vi "FreqTURBOGraph_ENGULx.vi"(0 "LCR-819 port name":refnum<visa-resource-name>="COM7") -> ()   [LabVIEW 2016]
doc: "The Basic Serial Read and Write example performs a Serial Port Read, a Serial Port Write, or a combination of these actions. The user selects the actions (read or write) on the front panel. If both are selected, the VI will write the data first, read data, and then close the VISA session that is opened to the port. This VI will wait until the specified number of bytes is received at the port. Only the number of bytes specified will be read.\n\nINSTRUCTIONS:\n1) Select the serial resource and configuration parameters (baud rate, data bits, parity, stop bits, flow control).\n2) Select the operations to be performed. \n3) Connect the serial port to your device. If no device is available, perform a loopback test by doing one of the following. Short pins 2 and 3 on a RS-232 cable or short pin 4 to pin 8 and pin 5 to pin 9 on a RS-485/422 cable. \n4) Run the VI to see the data read. (The \"read string\" will match the \"string to write\" if a loopback test was performed.)\n\nNote: The parameters set for the serial port must match the parameters of the connected instrument or device. In this example, the bytes to read parameter specifies the number of bytes that the serial port reads. If there were more bytes at the port than the number specified in bytes to read, those bytes would not be read. Also, if you specify to read more bytes than the number of bytes actually read, you might receive a timeout error message.\n\nOn the block diagram, the Configure Serial Port VI sets the configuration parameters. The front panel displays the controls used to configure the basic parameters, such as baud rate, data bits, and parity. Constants configure the other parameters the user probably does not need set. After the VISA Configure Serial Port VI opens the VISA session and configures the port, the VI passes the VISA resource name to other VIs that perform operations on that VISA resource. The VISA Write function sends a command to the serial device and the VISA Read function returns data based on the command. The VISA Close function then closes the reference to the serial device. It is important to close the reference; otherwise communication through with that port through protocols other than VISA might not be possible."
uses:
  <vilib>/Instr/_visa.llb/VISA Configure Serial Port (Instr).vi
panel:
  in  "STOP":bool
  out "Temperature, К":dbl
  out "Cole-Cole plot":cluster{dbl, dbl}[](graph)
  out "Frequency dependency of E' E\"":cluster{dbl, dbl, dbl}[](graph)
  out "Epsilon\"":dbl
  out "Epsilon'":dbl
  in  "Thickness, mm":dbl=1.75
  in  "Area, mm2":dbl=20.0
  in  "Comments":string="Sn2P2S6HighT\nS=20mm2 D=1.75mm\n"
  out "Data File":path
  in  "File name":path=path "proba.txt"
  out "Frequency, kHz":dbl
  out "Loss":dbl
  out "Capacity, F":dbl
  out "Current Frequency":string
  out "Frequency":string
  out "Data from LCR-meter":string
  out "Output":string
  # "LCR-819 Service information"
  # "Output Data File"
  # "Data from LCR-meter"
  # "Sample Size"
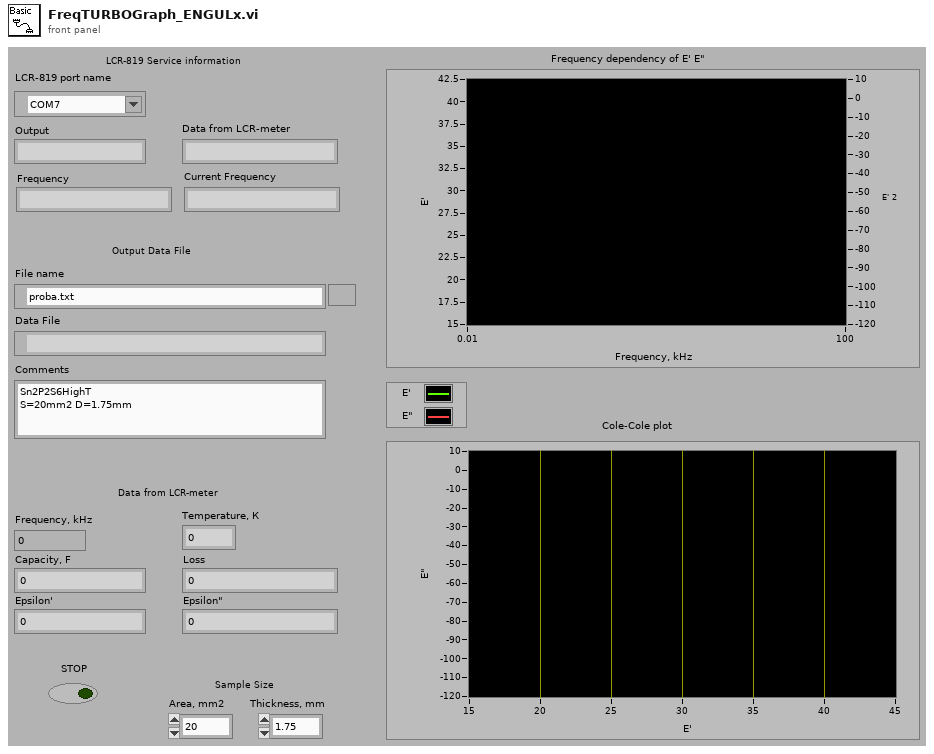
[diagram p1: front panel]
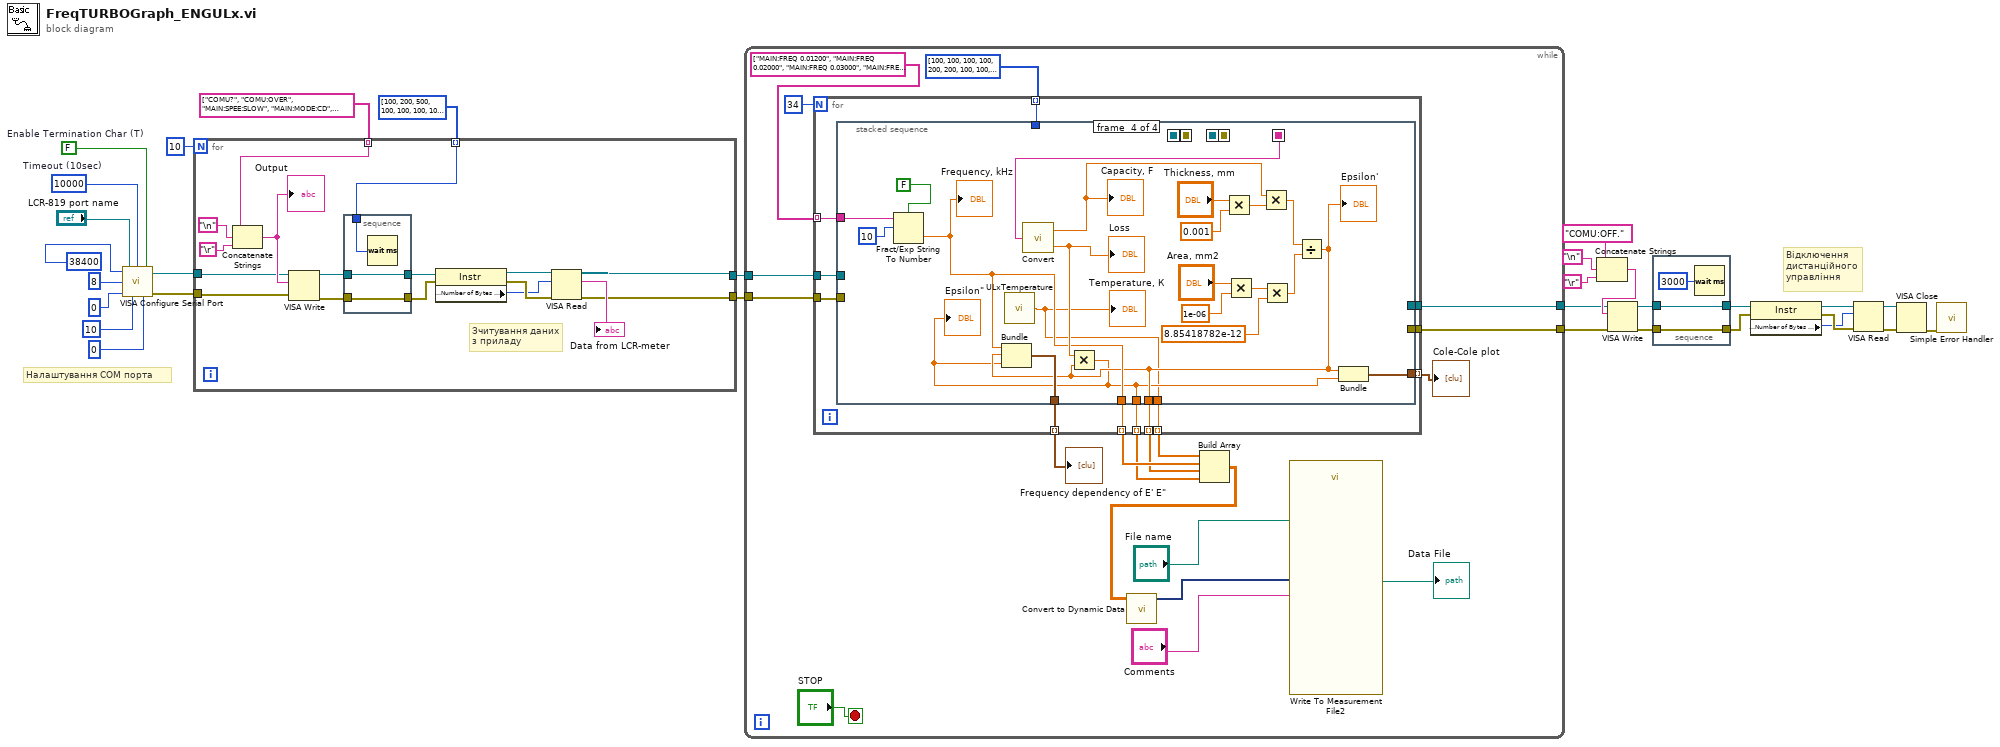
[diagram p0: block diagram]
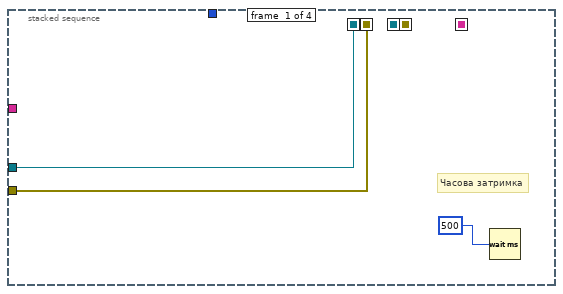
[diagram p2: hidden frame]
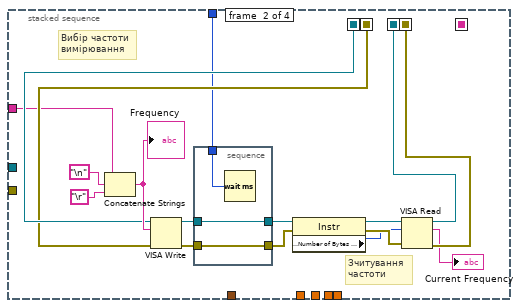
[diagram p3: hidden frame]
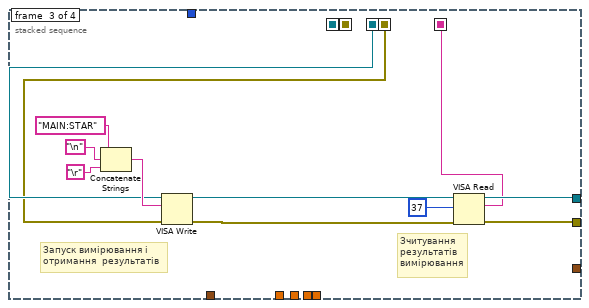
[diagram p4: hidden frame]
diagram:
  w29 = FALSE  # Enable Termination Char (T)
  w30 = u32 10000  # Timeout (10sec)
  # "Відключення дистанційного управління"
  # "Налаштування COM порта"
  n1 = call-poly "VISA Configure Serial Port"("VISA resource name"="LCR-819 port name", "timeout (10sec)"=w30, "Enable Termination\nChar (T)"=w29, "baud rate (9600)"=38400, "data bits (8)"=8, "parity (0:none)"=0, "stop bits (10: 1 bit)"=10, "flow control (0:none)"=0) -> ("VISA resource name out"=w24:refnum<visa-resource-name>, "error out"=w23:errorcluster)  [unwired: 6 in]
  n2 = for {
    N: 10 -> [_]
    tunnel: string[] ["COMU?", "COMU:OVER", "MAIN:SPEE:SLOW", "MAIN:MODE:CD", "MAIN:CIRC:PARA", "MAIN:TRIG:MANU", "MAIN:VOLT 1.250", "COMU:OFF.", "COMU?", "COMU:OVER", "", "", "", "", "", "", "", "", "", "", "", "", "", "", "", "", "", "", "", "", "", "", "", "", ""] -> [w37] mode=indexing
    tunnel: i32[] [100, 200, 500, 100, 100, 100, 100, 500, 200, 600, 0, 0, 0, 0, 0, 0, 0, 0, 0, 0, 0, 0, 0, 0, 0, 0, 0, 0, 0, 0, 0, 0, 0, 0, 0] -> [w36] mode=indexing
    tunnel: w24 -> [w35]
    tunnel: w23 -> [w34]
    tunnel: [w33] -> w4
    tunnel: [w32] -> w3
    # "Зчитування даних  з приладу"
    n3 = Concatenate Strings(w37, "\n", "\r") -> (w38:string)
    "Output" <- w38
    n4 = VISA Write(VISA resource name=w35, write buffer=w38, error in (no error)=w34) -> (VISA resource name out=w46:refnum<visa-resource-name>, error out=w48:errorcluster)  [unwired: 1 out]
    n5 = stacked-sequence {
      tunnel: w48 -> [w51]
      tunnel: [w51] -> w47
      tunnel: w46 -> [w50]
      tunnel: [w50] -> w45
      tunnel: w36 -> [w49]
      frame #0 {
        n6 = Wait (ms)(milliseconds to wait=w49) -> ()  [unwired: 1 out]
      }
    }
    n7 = property class="Instr"(reference=w45, error in=w47) -> (reference out=w44:refnum<visa-resource-name>, error out=w43:errorcluster, "Serial Settings:Number of Bytes at Serial Port"=w42:u32)
    n8 = VISA Read(VISA resource name=w44, byte count=w42, error in (no error)=w43) -> (VISA resource name out=w33:refnum<visa-resource-name>, read buffer=→"Data from LCR-meter":string, error out=w32:errorcluster)  [unwired: 1 out]
  }
  n9 = while {
    tunnel: w4 -> [w70]
    tunnel: w3 -> [w69]
    tunnel: [w68] -> w2
    tunnel: [w67] -> w1
    stop <- "STOP" stop-if-true
    n10 = for {
      N: 34 -> [_]
      tunnel: w70 -> [w82]
      tunnel: w69 -> [w81]
      tunnel: [w80] -> w68
      tunnel: [w79] -> w67
      tunnel: string[] ["MAIN:FREQ 0.01200", "MAIN:FREQ 0.02000", "MAIN:FREQ 0.03000", "MAIN:FREQ 0.04000", "MAIN:FREQ 0.06000", "MAIN:FREQ 0.06977", "MAIN:FREQ 0.07895", "MAIN:FREQ 0.09091", "MAIN:FREQ 0.10000", "MAIN:FREQ 0.20000", "MAIN:FREQ 0.30000", "MAIN:FREQ 0.40000", "MAIN:FREQ 0.50000", "MAIN:FREQ 0.60000", "MAIN:FREQ 0.69767", "MAIN:FREQ 0.80000", "MAIN:FREQ 0.89553", "MAIN:FREQ 1.00000", "MAIN:FREQ 2.00000", "MAIN:FREQ 3.00000", "MAIN:FREQ 4.00000", "MAIN:FREQ 5.00000", "MAIN:FREQ 6.00000", "MAIN:FREQ 6.66667", "MAIN:FREQ 7.50000", "MAIN:FREQ 8.57143", "MAIN:FREQ 10.0000", "MAIN:FREQ 20.0000", "MAIN:FREQ 28.5714", "MAIN:FREQ 33.3333", "MAIN:FREQ 40.0000", "MAIN:FREQ 50.0000"] -> [w78] mode=indexing
      tunnel: i32[] [100, 100, 100, 100, 200, 200, 100, 100, 100, 100, 100, 100, 100, 100, 100, 100, 200, 200, 100, 100, 100, 100, 100, 100, 100, 100, 100, 100, 100, 100, 100, 100, 100, 100] -> [w77] mode=indexing
      tunnel: [w76] -> w62 mode=indexing
      tunnel: [w75] -> w61 mode=indexing
      tunnel: [w74] -> w60 mode=indexing
      tunnel: [w73] -> w59 mode=indexing
      tunnel: [w72] -> w58 mode=indexing
      tunnel: [w71] -> w57 mode=indexing
      n11 = stacked-sequence {
        seq-local: [w85 _ _ _] -> [_ w92 _ _]
        seq-local: [w84 _ _ _] -> [_ w91 _ _]
        seq-local: [_ w90 _ _] -> [_ _ w113 _]
        seq-local: [_ w89 _ _] -> [_ _ w112 _]
        seq-local: [_ _ w109 _] -> [_ _ _ w138]
        tunnel: w82 -> [w85 _ _ _]
        tunnel: w81 -> [w84 _ _ _]
        tunnel: [_ _ w111 _] -> w80
        tunnel: [_ _ w110 _] -> w79
        tunnel: w78 -> [_ w87 _ w135]
        tunnel: w77 -> [_ w86 _ _]
        tunnel: [_ _ _ w123] -> w76
        tunnel: [_ _ _ w122] -> w75
        tunnel: [_ _ _ w118] -> w74
        tunnel: [_ _ _ w121] -> w73
        tunnel: [_ _ _ w120] -> w72
        tunnel: [_ _ _ w119] -> w71
        frame #0 {
          # "Часова затримка"
          n12 = Wait (ms)(milliseconds to wait=500) -> ()  [unwired: 1 out]
        }
        frame #1 {
          # "Вибір частоти вимірювання"
          # "Зчитування частоти"
          n13 = Concatenate Strings(w87, "\n", "\r") -> (w93:string)
          "Frequency" <- w93
          n14 = VISA Write(VISA resource name=w92, write buffer=w93, error in (no error)=w91) -> (VISA resource name out=w100:refnum<visa-resource-name>, error out=w102:errorcluster)  [unwired: 1 out]
          n15 = stacked-sequence {
            tunnel: w102 -> [w105]
            tunnel: [w105] -> w101
            tunnel: w100 -> [w104]
            tunnel: [w104] -> w99
            tunnel: w86 -> [w103]
            frame #0 {
              n16 = Wait (ms)(milliseconds to wait=w103) -> ()  [unwired: 1 out]
            }
          }
          n17 = property class="Instr"(reference=w99, error in=w101) -> (reference out=w98:refnum<visa-resource-name>, error out=w97:errorcluster, "Serial Settings:Number of Bytes at Serial Port"=w96:u32)
          n18 = VISA Read(VISA resource name=w98, byte count=w96, error in (no error)=w97) -> (VISA resource name out=w90:refnum<visa-resource-name>, read buffer=→"Current Frequency":string, error out=w89:errorcluster)  [unwired: 1 out]
        }
        frame #2 {
          # "Запуск вимірювання і отримання  результатів"
          # "Зчитування результатів вимірювання"
          n19 = Concatenate Strings("MAIN:STAR" ("string"), "\n", "\r") -> (w114:string)
          n20 = VISA Write(VISA resource name=w113, write buffer=w114, error in (no error)=w112) -> (VISA resource name out=w107:refnum<visa-resource-name>, error out=w106:errorcluster)  [unwired: 1 out]
          n21 = VISA Read(VISA resource name=w107, byte count=37, error in (no error)=w106) -> (VISA resource name out=w111:refnum<visa-resource-name>, read buffer=w109:string, error out=w110:errorcluster)  [unwired: 1 out]
        }
        frame #3 {
          n22 = Fract/Exp String To Number(use system decimal point (T)=FALSE, string=w135, offset=10) -> (number=w121:dbl)  [unwired: 1 in, 1 out]
          "Frequency, kHz" <- w121
          n23 = call "ULxTemperature.vi"() -> ("Temperature"=w118:dbl)
          "Temperature, К" <- w118
          n24 = call "Convert.vi"("Данные с прибора"=w138) -> ("Емкость"=w125:dbl, "Потери"=w124:dbl)
          "Capacity, F" <- w125
          "Loss" <- w124
          n25 = Multiply(x="Thickness, mm", y=0.001) -> (x*y=w132:dbl)
          n26 = Multiply(x="Area, mm2", y=1e-06) -> (x*y=w130:dbl)
          n27 = Multiply(x=w125, y=w132) -> (x*y=w133:dbl)
          n28 = Multiply(x=w130, y=8.85418782e-12) -> (x*y=w134:dbl)
          n29 = Divide(x=w133, y=w134) -> (x/y=w120:dbl)
          "Epsilon'" <- w120
          n30 = Multiply(x=w124, y=w120) -> (x*y=w119:dbl)
          "Epsilon\"" <- w119
          n31 = Bundle(w121, w120, w119) -> (w123:cluster{dbl, dbl, dbl})  [unwired: 1 in]
          n32 = Bundle(w120, w119) -> (w122:cluster{dbl, dbl})  [unwired: 1 in]
        }
      }
    }
    "Frequency dependency of E' E\"" <- w62
    "Cole-Cole plot" <- w61
    n33 = Build Array(w60, w59, w58, w57) -> (w53:dbl[][])
    n34 = call "Convert to Dynamic Data"("2D Array"=w53) -> ("Dynamic Data Type"=w52:dynamicdata)  [unwired: 3 in]
    n35 = call "Write To Measurement File2"("Signals"=w52, "Filename"="File name", "Comment"="Comments") -> ("Filename Out"=→"Data File":path)  [unwired: 14 in, 2 out]
  }
  n36 = Concatenate Strings("COMU:OFF." ("string"), "\n", "\r") -> (w12:string)
  n37 = VISA Write(VISA resource name=w2, write buffer=w12, error in (no error)=w1) -> (VISA resource name out=w20:refnum<visa-resource-name>, error out=w22:errorcluster)  [unwired: 1 out]
  n38 = stacked-sequence {
    tunnel: w22 -> [w141]
    tunnel: [w141] -> w21
    tunnel: w20 -> [w140]
    tunnel: [w140] -> w19
    frame #0 {
      n39 = Wait (ms)(milliseconds to wait=3000) -> ()  [unwired: 1 out]
    }
  }
  n40 = property class="Instr"(reference=w19, error in=w21) -> (reference out=w18:refnum<visa-resource-name>, error out=w17:errorcluster, "Serial Settings:Number of Bytes at Serial Port"=w16:u32)
  n41 = VISA Read(VISA resource name=w18, byte count=w16, error in (no error)=w17) -> (VISA resource name out=w11:refnum<visa-resource-name>, error out=w10:errorcluster)  [unwired: 2 out]
  n42 = VISA Close(VISA resource name=w11, error in (no error)=w10) -> (error out=w28:errorcluster)
  n43 = call <vilib>:"Simple Error Handler.vi"("error in (no error)"=w28) -> ()  [unwired: 4 in, 5 out]
